vi "RespiratoryControl.vi"(10 "Output Rate (ms)":u32=10 min=6 max=100000 step=1) -> ()   [LabVIEW 2019]
doc: "This VI is designed to output a sine wave with a DC offset of 2.5V and is especially intended for the USB-6008 and USB-6009. These devices are unique in the fact that they only support software timed analog output and their output range is 0V to 5V."
uses:
  <vilib>/Utility/error.llb/DialogType.ctl
  <vilib>/Analysis/baseanly.llb/Mean (DBL).vi
  <vilib>/ptbypt/NI_PtbyPt.lvlib
  <vilib>/Analysis/NI_AALBase.lvlib
panel:
  out "AIN2 2":dbl format="%.6f"
  in  "Expiration cmH2O":dbl(slide) scale=0.0..100.0
  in  "Inspiration Pause cmH2O":dbl(slide) scale=0.0..100.0
  in  "Inspiration Flow cmH2O":dbl(slide) scale=0.0..100.0
  in  "Rise time Seconds":dbl(slide)=0.01 min=0.01 max=0.5 scale=0.0..1.0
  in  "Inspiration Flow Percent":dbl(slide)=0.25 min=0.25 max=0.75 scale=0.0..1.0
  in  "Inspiration Period Percent":dbl(slide)=0.25 min=0.25 max=0.75 scale=0.0..1.0
  in  "stop":bool
  out "Error Message":string
  out "error out":errorcluster
  out "Output Data 2":dbl(graph)
  # "Timing Parameters"
  # "Pressure Parameters"
  # "Waveform Parameters"
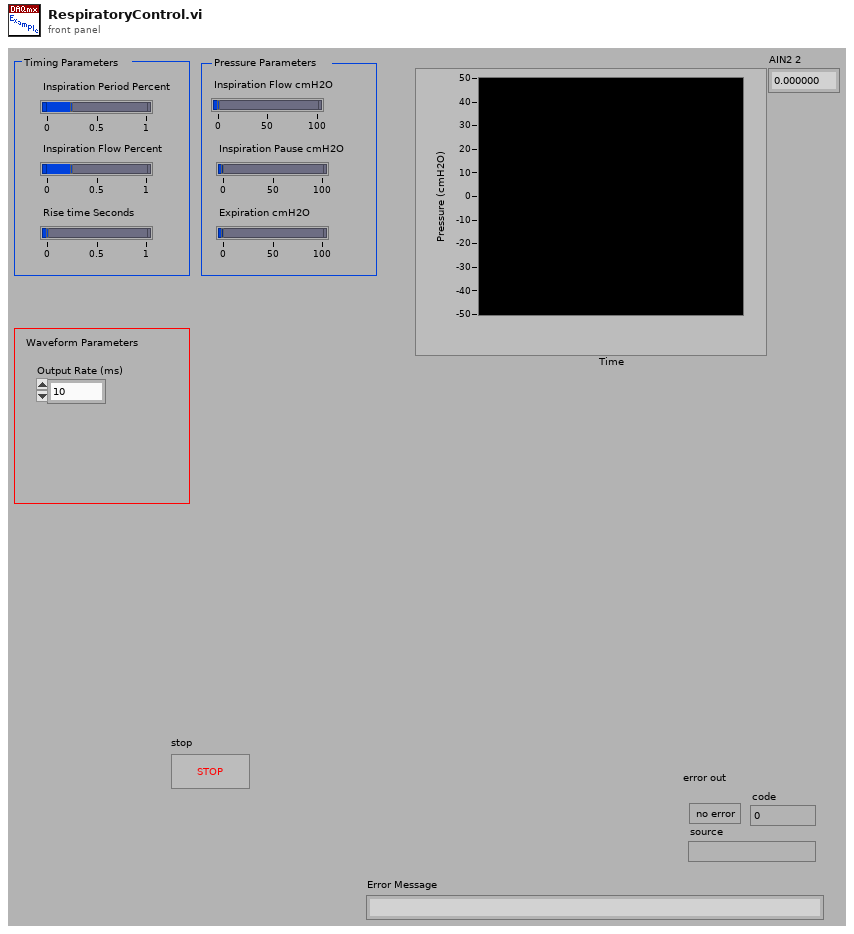
[diagram p1: front panel]
types:
  T1 = typedef "DialogType.ctl" = u16
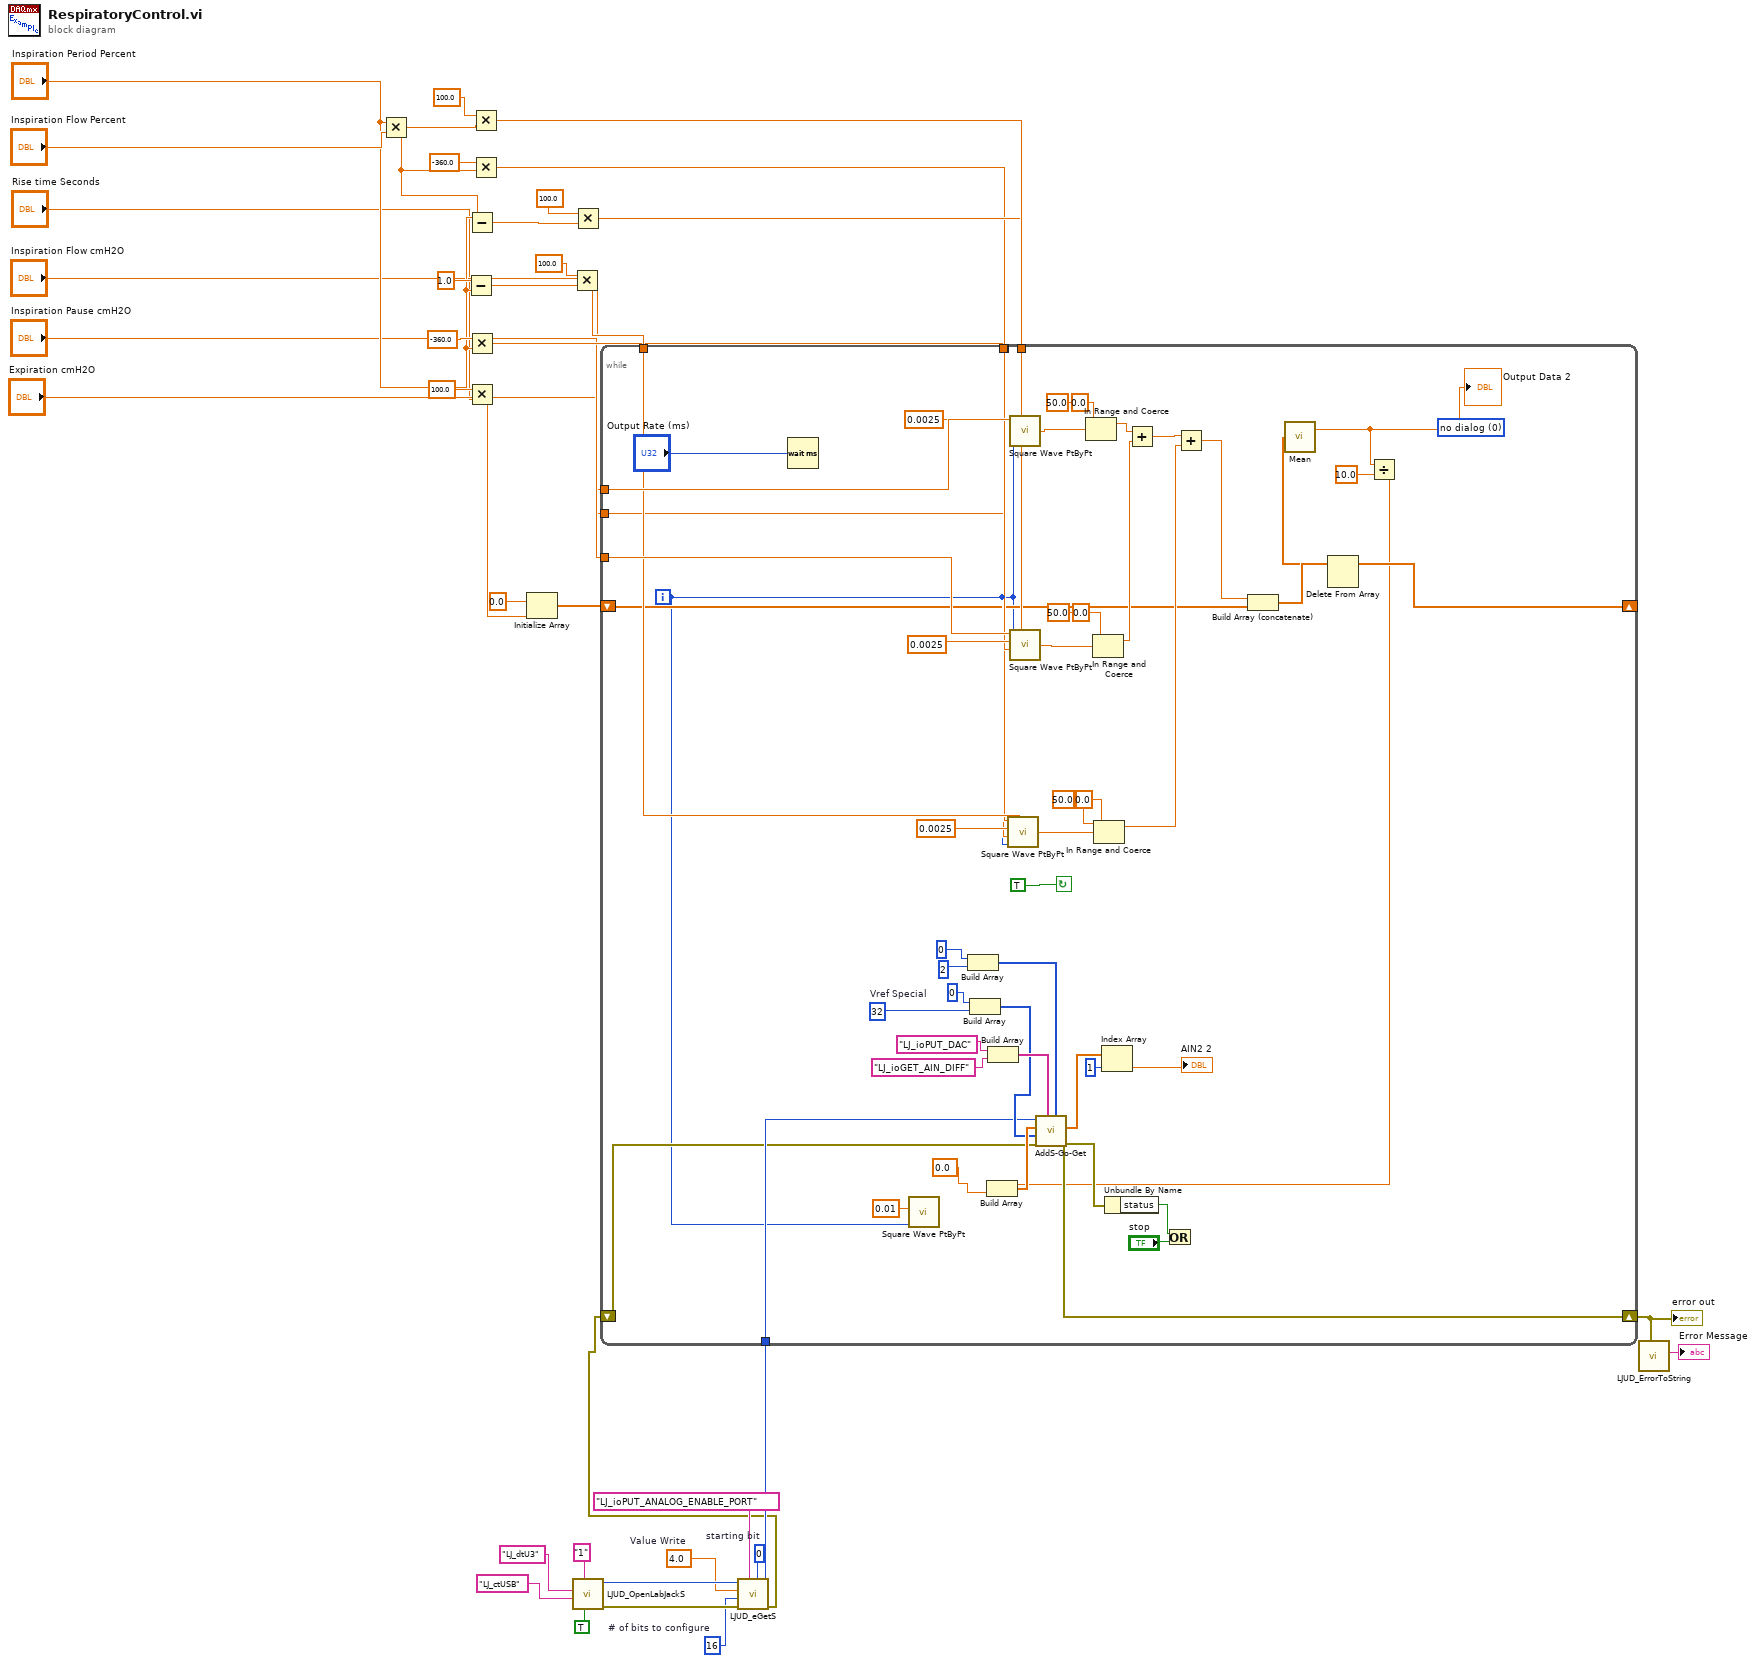
[diagram p0: block diagram]
diagram:
  w11 = 16  # # of bits to configure
  w13 = 0  # starting bit
  w14 = 4.0  # Value Write
  (unwired) T1 0 items=["no dialog", "OK message", "continue or stop message", "OK message + warnings", "continue/stop + warnings"] ("type of dialog (OK msg:1)")
  n1 = Multiply(x="Inspiration Period Percent", y="Inspiration Flow Percent") -> (x*y=w33:dbl)
  n2 = Subtract(x=1.0, y="Inspiration Period Percent") -> (x-y=w28:dbl)
  n3 = Subtract(x="Inspiration Period Percent", y=w33) -> (x-y=w36:dbl)
  n4 = Multiply(x=-360.0, y="Inspiration Period Percent") -> (x*y=w25:dbl)
  n5 = Multiply(x=100.0, y="Rise time Seconds") -> (x*y=w1:dbl)
  n6 = Multiply(x=100.0, y=w33) -> (x*y=w37:dbl)
  n7 = Multiply(x=-360.0, y=w33) -> (x*y=w31:dbl)
  n8 = Initialize Array(0.0 ("element"), w1) -> (w23:dbl[])
  n9 = Multiply(x=100.0, y=w28) -> (x*y=w27:dbl)
  n10 = Multiply(x=100.0, y=w36) -> (x*y=w34:dbl)
  n11 = call "LJUD_OpenLabJackS.vi"("FirstFound"=TRUE, "Address"="1", "ConnectionType"="LJ_ctUSB", "DeviceType"="LJ_dtU3") -> ("error out"=w15:errorcluster, "Handle"=w16:i32)  [unwired: 5 in, 1 out]
  n12 = call "LJUD_eGetS.vi"("Channel"=w13, "IOType"="LJ_ioPUT_ANALOG_ENABLE_PORT", "error in"=w15, "x1"=w11, "Value Write"=w14, "Handle In"=w16) -> ("error out"=w9:errorcluster, "Handle Out"=w10:i32)  [unwired: 3 in, 1 out]
  n13 = while {
    tunnel: "Inspiration Flow cmH2O" -> [w90]
    tunnel: "Inspiration Pause cmH2O" -> [w87]
    tunnel: w37 -> [w86]
    tunnel: w34 -> [w85]
    tunnel: w31 -> [w84]
    tunnel: w27 -> [w72]
    tunnel: "Expiration cmH2O" -> [w71]
    tunnel: w25 -> [w69]
    shift-right: [w63] -> _
    shift-left: w23 -> [w64]
    tunnel: w10 -> [w46]
    shift-right: [w44] -> w8
    shift-left: w9 -> [w45]
    i -> [w43]
    stop <- TRUE continue-if-true
    w50 = 32  # Vref Special
    n14 = Wait (ms)(milliseconds to wait="Output Rate (ms)") -> ()  [unwired: 1 out]
    n15 = call <vilib>:"Square Wave PtByPt.vi"("frequency"=0.01, "time"=w43) -> ()  [unwired: 3 in, 1 out]
    n16 = Build Array(0, 2) -> (w61:i32[])
    n17 = Build Array(0, w50) -> (w49:i32[])
    n18 = Build Array("LJ_ioPUT_DAC" ("IOType"), "LJ_ioGET_AIN_DIFF" ("IOType")) -> (w62:string[])
    n19 = call <vilib>:"Square Wave PtByPt.vi"("amplitude"=w71, "frequency"=0.0025, "phase"=w69, "time"=w43, "duty cycle (%)"=w72) -> ("square wave"=w73:dbl)
    n20 = call <vilib>:"Square Wave PtByPt.vi"("amplitude"=w90, "frequency"=0.0025, "time"=w43, "duty cycle (%)"=w86) -> ("square wave"=w83:dbl)  [unwired: 1 in]
    n21 = call <vilib>:"Square Wave PtByPt.vi"("amplitude"=w87, "frequency"=0.0025, "phase"=w84, "time"=w43, "duty cycle (%)"=w85) -> ("square wave"=w81:dbl)
    n22 = In Range and Coerce(upper limit=50.0, x=w83, lower limit=0.0) -> (coerced(x)=w80:dbl)  [unwired: 1 out]
    n23 = In Range and Coerce(upper limit=50.0, x=w81, lower limit=0.0) -> (coerced(x)=w79:dbl)  [unwired: 1 out]
    n24 = In Range and Coerce(upper limit=50.0, x=w73, lower limit=0.0) -> (coerced(x)=w68:dbl)  [unwired: 1 out]
    n25 = Add(x=w80, y=w79) -> (x+y=w67:dbl)
    n26 = Add(x=w67, y=w68) -> (x+y=w66:dbl)
    n27 = Build Array (concatenate)(w66, w64) -> (w65:dbl[])
    n28 = Delete From Array(array=w65) -> (array with subset deleted=w63:dbl[])  [unwired: 2 in, 1 out]
    n29 = call-poly <vilib>:"Mean.vi"("X"=w63) -> ("mean"=w41:dbl)  [unwired: 1 out]
    "Output Data 2" <- w41
    n30 = Divide(x=w41, y=10.0) -> (x/y=w39:dbl)
    n31 = Build Array(w39, 0.0 ("Input Element")) -> (w60:dbl[])
    n32 = call "AddS-Go-Get.vi"("Channels"=w61, "IOTypes"=w62, "error in"=w45, "x1"=w49, "Values Write"=w60, "Handle In"=w46) -> ("error out"=w44:errorcluster, "Values Read"=w54:dbl[])  [unwired: 3 in, 1 out]
    n33 = Index Array(array=w54, index=1 ("Index")) -> (element=→"AIN2 2":dbl)
    n34 = Unbundle By Name(w44) -> ("status"=w52:bool)
    n35 = Or(x=w52, y="stop") -> ()  [unwired: 1 out]
  }
  "error out" <- w8
  n36 = call "LJUD_ErrorToString.vi"("error in"=w8) -> ("String"=→"Error Message":string)  [unwired: 10 in]
